vi "Get FIFO Register Bus.vi"(2 "reference fpga":refnum<class "niUSRP Reference FPGA v1.lvclass">) -> (4 "fifo register bus":refnum<class "niInstr FIFO Register Bus v1 FPGA.lvclass">)   [LabVIEW 2025, in "niUSRP Reference FPGA v1.lvclass"]
uses:
  niUSRP Reference FPGA v1.lvclass
  <instrlib>/_niInstr/FIFO Register Bus/v1/FPGA/niInstr FIFO Register Bus v1 FPGA.lvclass
  niUSRP Reference FPGA v1.lvclass/niUSRP Reference FPGA v1.ctl
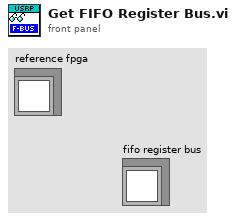
[diagram p1: front panel]
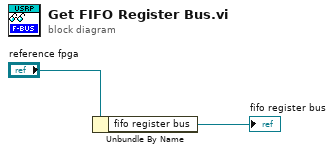
[diagram p0: block diagram]
diagram:
  n1 = Unbundle By Name("reference fpga") -> ("fifo register bus"=→"fifo register bus":refnum<class "niInstr FIFO Register Bus v1 FPGA.lvclass">)
